vi "Convert Variant To Error.vi"(10 "error in (no error)":errorcluster, 11 "Variant":variant) -> (2 "error out":errorcluster, 3 "Error":errorcluster)   [LabVIEW 2020, in "RTAF.lvlib"]
uses:
  RTAF.lvlib
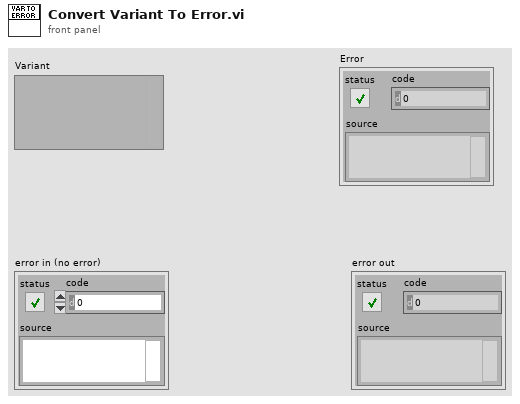
[diagram p1: front panel]
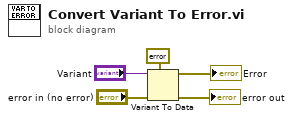
[diagram p0: block diagram]
diagram:
  n1 = Variant To Data(error in="error in (no error)", type=errorcluster {"status"=FALSE, "code"=0, "source"=""}, Variant="Variant") -> (data=→"Error":errorcluster, error out=→"error out":errorcluster)
